vi "Datasocket(Sin)客户机.vi"() -> ()   [LabVIEW 2017]
panel:
  out "URL":string
  in  "停止":bool
  out "波形图":dbl[](graph)
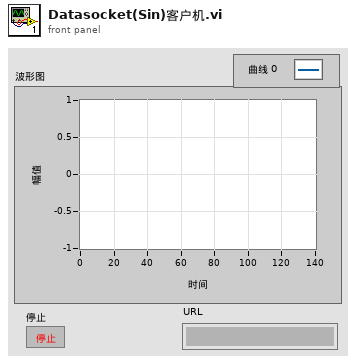
[diagram p1: front panel]
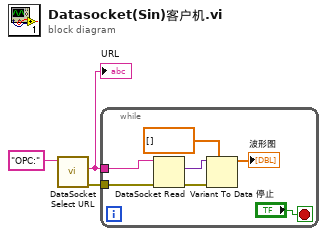
[diagram p0: block diagram]
diagram:
  n1 = call <vilib>:"DataSocket Select URL.vi"("StartURL (empty)"="OPC:") -> ("error out"=w1:errorcluster, "URL"=w2:string)  [unwired: 8 in, 1 out]
  "URL" <- w2
  n2 = while {
    tunnel: w2 -> [w10]
    tunnel: w1 -> [w9]
    stop <- "停止" stop-if-true
    n3 = DataSocket Read(8:w9, 11:w10) -> (0:w7:errorcluster, 2:w8:variant)  [unwired: 3 in, 5 out]
    n4 = Variant To Data(error in=w7, type=dbl[] [], Variant=w8) -> (data=→"波形图":dbl[])  [unwired: 1 out]
  }
